vi "MultiLineString_Delete.vi"(0 "reference in":refnum<class "MultiLineString.lvclass">, 5 "error in (no error)":errorcluster) -> (14 "reference out":refnum<class "MultiLineString.lvclass">, 15 "# of objects":i32, 19 "error out":errorcluster)   [LabVIEW 2020, in "MultiLineString.lvclass"]
doc: "Deletes a MultiLineString object created with the MultiLineString new VI and returns the contents of the object.\n\n[GOOP 2.0.15]"
uses:
  <resource>/Framework/Providers/Open_GDS/UML/MultiLineString_class/MultiLineString.lvclass
  <vilib>/addons/_goop3.llb/3GOOPStates.ctl
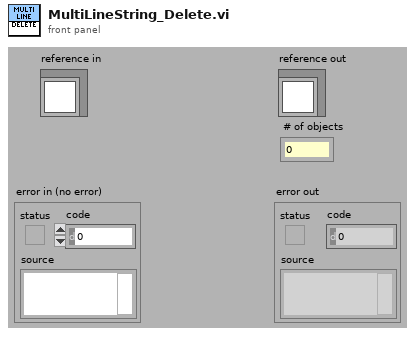
[diagram p1: front panel]
types:
  T1 = typedef "3GOOPStates.ctl" = enum16{"Set", "Get", "New", "Delete", "Clear", "Test and get", "Unlock data", "Information", "Look up existing", "New or look up existing", "Test and get shared", "Get shared", "Set shared", "Unlock shared", "Find dynamic method", "Register dynamic method", "Preload dynamic method", "Probe", "Cast to more generic", "Cast to more specific"}
  T2 = typedef "MultiLineString.lvclass/ObjectReference.ctl" = refnum<k1>
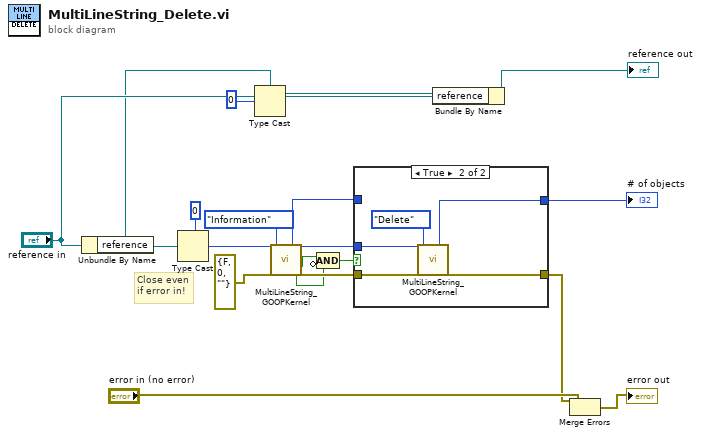
[diagram p0: block diagram]
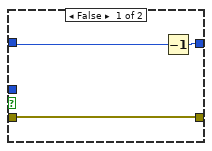
[diagram p2: hidden frame]
diagram:
  # "Close even\nif error in!"
  n1 = Unbundle By Name("reference in") -> ("reference"=w3:T2)
  n2 = Type Cast(type=0, x=w3) -> (*(type *) &x=w14:i32)
  n3 = Type Cast(type=w3, x=0) -> (*(type *) &x=w2:T2)
  n4 = call <resource>:"MultiLineString_GOOPKernel.vi"("Ref in"=w14, "error in (no error)"=errorcluster {"status"=FALSE, "code"=0, "source"=""}, "Action"=3GOOPStates."Information") -> ("# of objects"=w7:i32, "IsSubclass?"=w9:bool, "Ref out"=w13:i32, "Exists?"=w10:bool, "error out"=w12:errorcluster)  [unwired: 12 in, 8 out]
  n5 = Compound Arithmetic op=AND(w10, invert w9) -> (w8:bool)
  n6 = case shown="True" w8 {
    tunnel: w13 -> [_ w27]
    tunnel: [w20 w26] -> w16
    tunnel: [w22 w24] -> w15
    tunnel: w12 -> [w20 w25]
    tunnel: w7 -> [w21 _]
    frame False {
      n7 = Decrement(x=w21) -> (x-1=w22:i32)
    }
    frame True {
      n8 = call <resource>:"MultiLineString_GOOPKernel.vi"("Ref in"=w27, "error in (no error)"=w25, "Action"=3GOOPStates."Delete") -> ("# of objects"=w24:i32, "error out"=w26:errorcluster)  [unwired: 12 in, 11 out]
    }
  }
  "# of objects" <- w15
  n9 = Bundle By Name(cluster="reference in", "reference"=w2) -> (→"reference out":refnum<class "MultiLineString.lvclass">)
  n10 = Merge Errors("error in (no error)", w16) -> (→"error out":errorcluster)
